vi "GetTempsRtd2wh.vi"() -> (4 "Temperatures":dbl[](array[numeric]), 6 "Variables":string[](array[string])=["Tifd", "Tvlna", "Thlna", "Thcirc", "Tvcirc", "Tsg", "Tinamb", "Toutamb", "Tateamp", "Tatedelay", "Te4418b", "Tvdumload", "Thdumload", "Tklystron", "Trxbox", "Tspare1", "Tspare2"], 8 "Temperature String":string, 15 "Error out":errorcluster)   [LabVIEW 2009]
panel:
  in  "Instrument":T1(ring)=enum."34980a"
  # "IFD"
  # "VLNA"
  # "HLNA"
  # "H Circ"
  # "V Circ"
  # "Siggen"
  # "Inside"
  # "Outside"
  # "ATE Amp"
  # "ATE Delay"
  # "TOF Pwr"
  # "V Dummy"
  # "H Dummy"
  # "Klystron"
  # "Rx Box"
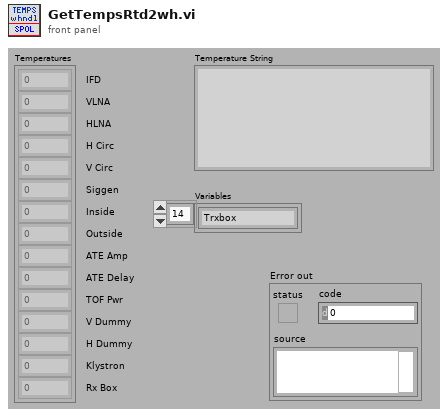
[diagram p1: front panel]
types:
  T1 = enum16{"N1911A", "Siggen", "34980a", "E4418B", "Rvp8"}
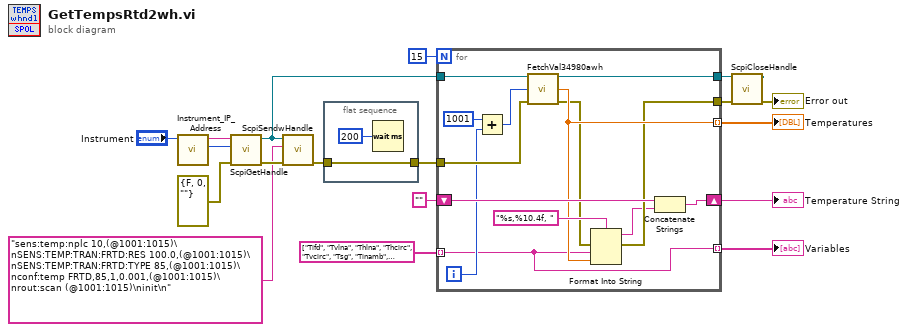
[diagram p0: block diagram]
diagram:
  n1 = call "Instrument_IP_Address.vi"("Instrument"="Instrument") -> ("Port"=w16:u16, "IP Address"=w17:string)  [unwired: 9 in]
  n2 = call "ScpiGetHandle.vi"("error in (no error)"=errorcluster {"status"=FALSE, "code"=0, "source"=""}, "TCP port"=w16, "IP Address"=w17) -> ("Error out"=w14:errorcluster, "connection ID"=w9:refnum<k5>)  [unwired: 6 in]
  n3 = call "ScpiSendwHandle.vi"("error in (no error)"=w14, "Command"="sens:temp:nplc 10,(@1001:1015)\nSENS:TEMP:TRAN:FRTD:RES 100.0,(@1001:1015)\nSENS:TEMP:TRAN:FRTD:TYPE 85,(@1001:1015)\nconf:temp FRTD,85,1,0.001,(@1001:1015)\nrout:scan (@1001:1015)\ninit\n" ("SCPI command"), "connection ID"=w9) -> ("error out"=w12:errorcluster)  [unwired: 7 in, 1 out]
  n4 = flat-sequence {
    tunnel: w12 -> [w19]
    tunnel: [w19] -> w10
    frame #0 {
      n5 = Wait (ms)(milliseconds to wait=u32 200) -> ()  [unwired: 1 out]
    }
  }
  n6 = for {
    N: 15 -> [_]
    tunnel: w10 -> [w32]
    tunnel: [w31] -> w7
    tunnel: [w24] -> w6
    tunnel: w9 -> [w30]
    tunnel: [w26] -> w8 mode=indexing
    tunnel: string[] ["Tifd", "Tvlna", "Thlna", "Thcirc", "Tvcirc", "Tsg", "Tinamb", "Toutamb", "Tateamp", "Tatedelay", "Te4418b", "Tvdumload", "Thdumload", "Tklystron", "Trxbox", "Spare1", "Spare2"] -> [w21] mode=indexing
    shift-right: [w28] -> w2
    shift-left: "" -> [w29]
    tunnel: [w21] -> w1 mode=indexing
    i -> [w22]
    n7 = Add(x=1001 ("Circuit ID"), y=w22) -> (x+y=w33:i32)
    n8 = call "FetchVal34980awh.vi"("connection ID In"=w30, "Circuit ID"=w33, "error in (no error)"=w32) -> ("connection ID Out"=w31:refnum<k5>, "Value"=w26:dbl, "Error out"=w25:errorcluster)  [unwired: 10 in]
    n9 = Format Into String(format string="%s,%10.4f, ", error in=w25, w21, w26) -> (resulting string=w23:string, error out=w24:errorcluster)  [unwired: 1 in]
    n10 = Concatenate Strings(w29, w23) -> (w28:string)
  }
  "Temperatures" <- w8
  "Temperature String" <- w2
  "Variables" <- w1
  n11 = call "ScpiCloseHandle.vi"("error in (no error)"=w6, "connection ID"=w7) -> ("Error out"=→"Error out":errorcluster)  [unwired: 8 in]
